vi "Pos_Select Random Box Position.vi"(7 "Work Space":T1, 8 "Error":errorcluster, 9 "Min Border":i16=5, 11 "Window Bounds":T1) -> (0 "Error Out":errorcluster, 3 "Window Bounds Out":T1)   [LabVIEW 2015]
uses:
  <vilib>/Utility/miscctls.llb/LVRectTypeDef.ctl
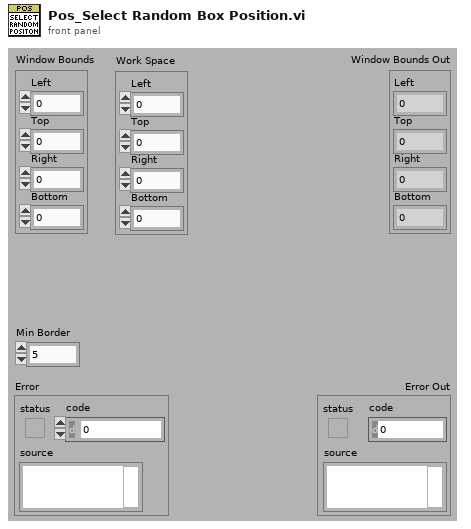
[diagram p1: front panel]
types:
  T1 = typedef "LVRectTypeDef.ctl" = cluster{"Left":i16, "Top":i16, "Right":i16, "Bottom":i16}
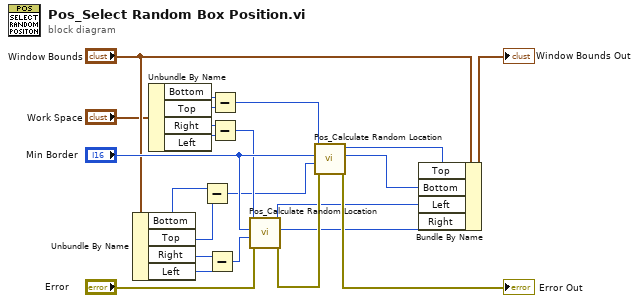
[diagram p0: block diagram]
diagram:
  n1 = Unbundle By Name("Window Bounds") -> ("Bottom"=w5:i16, "Top"=w6:i16, "Right"=w19:i16, "Left"=w18:i16)
  n2 = Unbundle By Name("Work Space") -> ("Bottom"=w15:i16, "Top"=w14:i16, "Right"=w12:i16, "Left"=w13:i16)
  n3 = Subtract(x=w5, y=w6) -> (x-y=w7:i16)
  n4 = Subtract(x=w19, y=w18) -> (x-y=w8:i16)
  n5 = Subtract(x=w15, y=w14) -> (x-y=w9:i16)
  n6 = Subtract(x=w12, y=w13) -> (x-y=w10:i16)
  n7 = call "Pos_Calculate Random Location.vi"("Error"="Error", "Window Size"=w8, "Border"="Min Border", "Max Size"=w10) -> ("Error Out"=w23:errorcluster, "Bottom Right Out"=w2:i16, "Top Left Out"=w4:i16)  [unwired: 5 in]
  n8 = call "Pos_Calculate Random Location.vi"("Error"=w23, "Window Size"=w7, "Border"="Min Border", "Max Size"=w9) -> ("Error Out"=→"Error Out":errorcluster, "Bottom Right Out"=w1:i16, "Top Left Out"=w3:i16)  [unwired: 5 in]
  n9 = Bundle By Name(cluster="Window Bounds", "Top"=w3, "Bottom"=w1, "Left"=w4, "Right"=w2) -> (→"Window Bounds Out":T1)
